vi "Pre Launch Init.vi"(11 "Module in":refnum<class "Module.lvclass">) -> (0 "error out":errorcluster, 3 "Module out":refnum<class "Module.lvclass">)   [LabVIEW 2025, in "Module.lvlib" / "Module.lvclass"]
doc: "<p>(<strong>Filename</strong>: <span class=\"dnl\">Actor Framework.lvlib:Actor.lvclass:Pre Launch Init.vi</span>)</p>\n<p>Defines behavior that occurs after the <a href=\"nihelplauncher://docs/csh?context=lvcore_lvcomm_af_launch_nested_actor\">Launch Nested Actor</a> method is invoked but before the actor's Actor Core method begins running.</p>\n<p>By default, this method does nothing. A descendant class may override it to define behavior.</p>"
uses:
  Module.lvclass
  Msg&Data.ctl
  Msg.ctl
  <vilib>/ActorFramework/Actor/Actor.lvclass
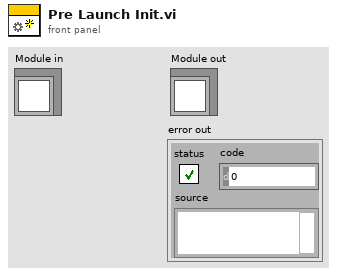
[diagram p1: front panel]
types:
  T1 = typedef "Msg&Data.ctl" = cluster{"Msg":T2, "Data":variant}
  T2 = typedef "Msg.ctl" = string
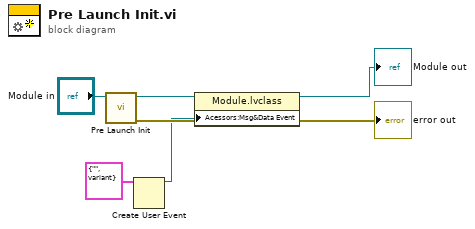
[diagram p0: block diagram]
diagram:
  n1 = call-parent "Pre Launch Init.vi"("Actor in"="Module in") -> ("error out"=→"error out":errorcluster, "Actor out"=w5:refnum<class "Module.lvclass">)  [unwired: 9 in]
  n2 = Create User Event(user event datatype=T1 {"Msg"="", "Data"=variant} ("Msg&Data")) -> (user event=w1:refnum<user-event>)  [unwired: 1 in, 1 out]
  n3 = property class="Module.lvclass"(reference=w5, "Acessors:Msg&Data Event"=w1) -> (reference out=→"Module out":refnum<class "Module.lvclass">)  [unwired: 1 in, 1 out]
